vi "Destroy Helper Loop Events.vi"(11 "Acquisition in":refnum<class "Acquisition.lvclass">) -> ()   [LabVIEW 2018, in "Acquisition.lvlib" / "Acquisition.lvclass"]
uses:
  Acquisition.lvclass
  Acquisition.lvclass/Acquisition.ctl
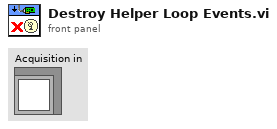
[diagram p1: front panel]
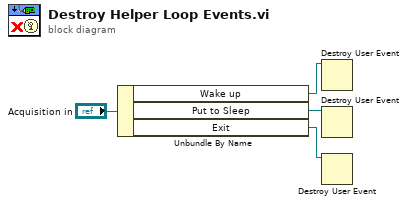
[diagram p0: block diagram]
diagram:
  n1 = Unbundle By Name("Acquisition in") -> ("Wake up"=w1:refnum<user-event>, "Put to Sleep"=w2:refnum<user-event>, "Exit"=w3:refnum<user-event>)
  n2 = Destroy User Event(user event=w1) -> ()  [unwired: 1 in, 1 out]
  n3 = Destroy User Event(user event=w2) -> ()  [unwired: 1 in, 1 out]
  n4 = Destroy User Event(user event=w3) -> ()  [unwired: 1 in, 1 out]
